vi "Check for Definition.vi"(8 "error in (no error)":errorcluster, 11 "Definition Name":string) -> (0 "error out":errorcluster, 3 "Found?":bool)   [LabVIEW 2020, in "JSON Schema Generator.lvlib"]
uses:
  JSON Schema Generator.lvlib
  Defintion FGV Actions.ctl
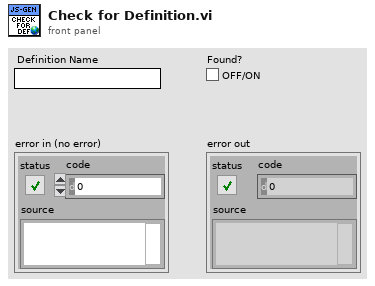
[diagram p1: front panel]
types:
  T1 = typedef "JSON Schema Generator.lvlib/Defintion FGV Actions.ctl" = enum16{"Create Defs", "Update Defs", "Get all Defs", "Get Def"}
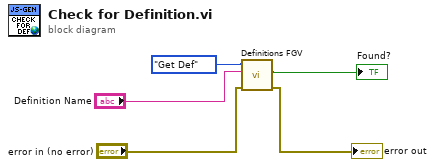
[diagram p0: block diagram]
diagram:
  n1 = call "Definitions FGV.vi"("error in (no error)"="error in (no error)", "Definition Name"="Definition Name", "Action"=Defintion_FGV_Actions."Get Def") -> ("error out"=→"error out":errorcluster, "Found?"=→"Found?":bool)  [unwired: 6 in, 1 out]
